vi "UpdateMetricCacheUnits.vi"(8 "error in (no error)":errorcluster, 9 "properties":T1[](array[typedef]), 10 "metric definition instance id":string, 11 "metric cache in":variant) -> (0 "error out":errorcluster, 1 "properties out":T1[](array[typedef]), 3 "metric cache out":variant)   [LabVIEW 2017, in "AnalysisHelper.lvlib"]
uses:
  <vilib>/addons/InsightCM/Utilities/Analysis/Shared/AnalysisHelper.lvlib
  <vilib>/addons/InsightCM/MessageBus/Base/controls/KeyValuePair.ctl
  <vilib>/addons/InsightCM/Utilities/PropertyHelpers/PropertyHelpers.lvlib
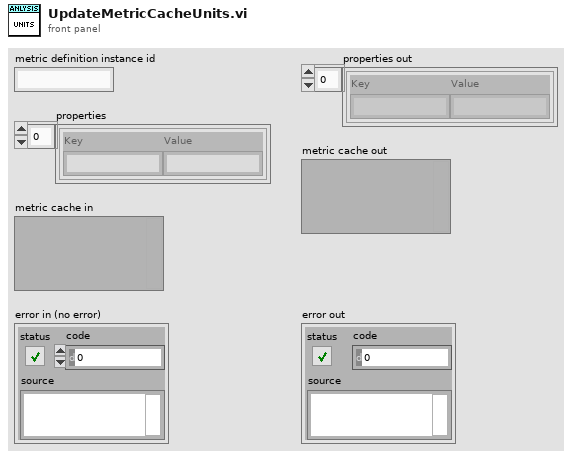
[diagram p1: front panel]
types:
  T1 = typedef "KeyValuePair.ctl" = cluster{"Key":string, "Value":string}
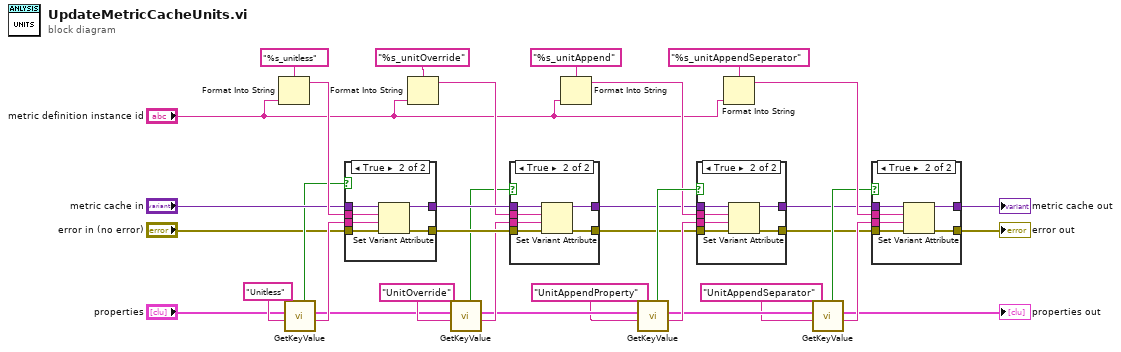
[diagram p0: block diagram]
diagram:
  n1 = Format Into String(format string="%s_unitless", "metric definition instance id") -> (resulting string=w36:string)  [unwired: 2 in, 1 out]
  n2 = call <vilib>:"GetKeyValue.vi"("key"="Unitless", "key value pairs"="properties") -> ("value"=w27:string, "key value pairs out"=w23:T1[], "found"=w28:bool)  [unwired: 7 in]
  n3 = case shown="True" w28 {
    tunnel: "metric cache in" -> [w38 w44]
    tunnel: [w38 w43] -> w35
    tunnel: "error in (no error)" -> [w37 w42]
    tunnel: [w37 w41] -> w24
    tunnel: w36 -> [_ w40]
    tunnel: w27 -> [_ w39]
    frame False {
    }
    frame True {
      n4 = Set Variant Attribute(Variant=w44, name=w40, value=w39, error in=w42) -> (Variant out=w43:variant, error out=w41:errorcluster)  [unwired: 1 out]
    }
  }
  n5 = Format Into String(format string="%s_unitOverride", "metric definition instance id") -> (resulting string=w32:string)  [unwired: 2 in, 1 out]
  n6 = call <vilib>:"GetKeyValue.vi"("key"="UnitOverride", "key value pairs"=w23) -> ("value"=w21:string, "key value pairs out"=w9:T1[], "found"=w22:bool)  [unwired: 7 in]
  n7 = case shown="True" w22 {
    tunnel: [w46 w50] -> w13
    tunnel: w35 -> [w46 w49]
    tunnel: [w45 w51] -> w14
    tunnel: w24 -> [w45 w52]
    tunnel: w32 -> [_ w48]
    tunnel: w21 -> [_ w47]
    frame False {
    }
    frame True {
      n8 = Set Variant Attribute(Variant=w49, name=w48, value=w47, error in=w52) -> (Variant out=w50:variant, error out=w51:errorcluster)  [unwired: 1 out]
    }
  }
  n9 = Format Into String(format string="%s_unitAppend", "metric definition instance id") -> (resulting string=w18:string)  [unwired: 2 in, 1 out]
  n10 = call <vilib>:"GetKeyValue.vi"("key"="UnitAppendProperty", "key value pairs"=w9) -> ("value"=w20:string, "key value pairs out"=w8:T1[], "found"=w19:bool)  [unwired: 7 in]
  n11 = case shown="True" w19 {
    tunnel: [w54 w58] -> w12
    tunnel: w13 -> [w54 w57]
    tunnel: [w53 w59] -> w11
    tunnel: w14 -> [w53 w60]
    tunnel: w18 -> [_ w56]
    tunnel: w20 -> [_ w55]
    frame False {
    }
    frame True {
      n12 = Set Variant Attribute(Variant=w57, name=w56, value=w55, error in=w60) -> (Variant out=w58:variant, error out=w59:errorcluster)  [unwired: 1 out]
    }
  }
  n13 = Format Into String(format string="%s_unitAppendSeperator", "metric definition instance id") -> (resulting string=w17:string)  [unwired: 2 in, 1 out]
  n14 = call <vilib>:"GetKeyValue.vi"("key"="UnitAppendSeparator", "key value pairs"=w8) -> ("value"=w15:string, "key value pairs out"=→"properties out":T1[], "found"=w16:bool)  [unwired: 7 in]
  n15 = case shown="True" w16 {
    tunnel: [w62 w66] -> w1
    tunnel: w12 -> [w62 w65]
    tunnel: [w61 w67] -> w2
    tunnel: w11 -> [w61 w68]
    tunnel: w17 -> [_ w64]
    tunnel: w15 -> [_ w63]
    frame False {
    }
    frame True {
      n16 = Set Variant Attribute(Variant=w65, name=w64, value=w63, error in=w68) -> (Variant out=w66:variant, error out=w67:errorcluster)  [unwired: 1 out]
    }
  }
  "error out" <- w2
  "metric cache out" <- w1
